vi "limelightDrive.vi"(10 "reinitialize? (F)":bool) -> (0 "Valid Track":bool=TRUE, 2 "Turn Output":dbl=0.011269776979651982)   [LabVIEW 2018]
uses:
  <vilib>/addons/control/pid/pid.llb/PID (DBL).vi
  <vilib>/addons/control/pid/NI_PID_pid.lvlib
panel:
  in  "output range":cluster{"output high":dbl, "output low":dbl}={"output high"=0.6, "output low"=-0.6}
  out "PID Output":dbl(graph)=0.011269776979651982
  in  "PID gains":T1={"proportional gain (Kc)"=0.013, "integral time (Ti, min)"=0.2, "derivative time (Td, min)"=0.0009} {"derivative time (Td, min)" format="%.4f"; "integral time (Ti, min)" format="%.3f"; "proportional gain (Kc)" format="%.3f"}
  out "Camera X":cluster{"setpoint":dbl, "Double":dbl}(graph)={"setpoint"=0.0, "Double"=-0.6907806396484375}
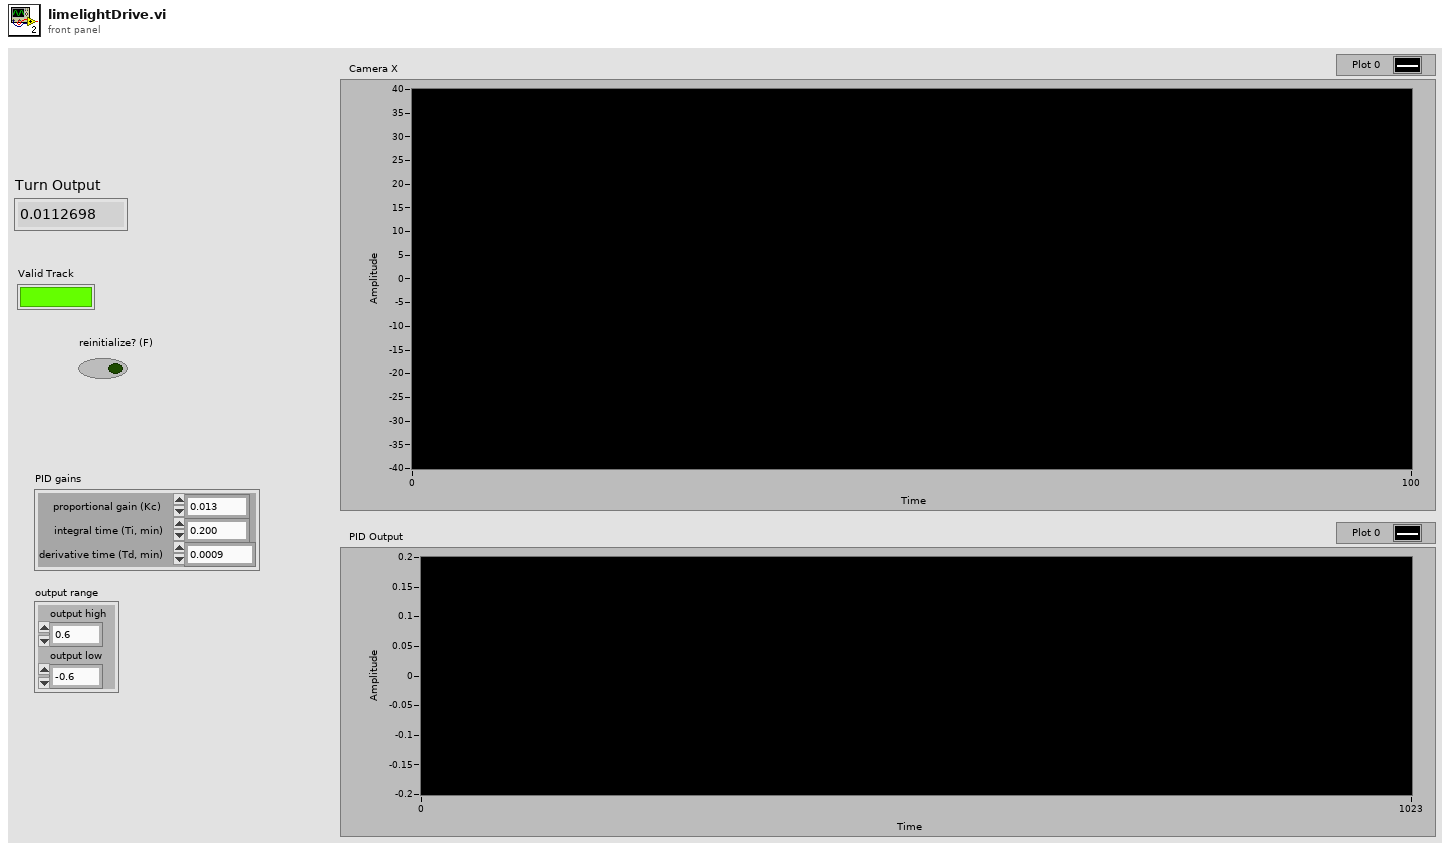
[diagram p1: front panel]
types:
  T1 = cluster{"proportional gain (Kc)":dbl, "integral time (Ti, min)":dbl, "derivative time (Td, min)":dbl}
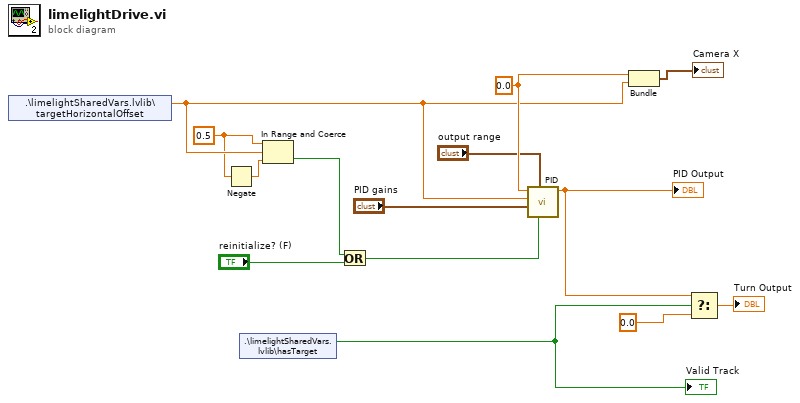
[diagram p0: block diagram]
diagram:
  w6 = 0.5 ("upper limit")
  w14 = 0.0 ("setpoint")
  n1 = shared-variable ".\\limelightSharedVars.lvlib\\targetHorizontalOffset"() -> (w8:dbl)  [unwired: 1 in, 1 out]
  n2 = Negate(x=w6) -> (-x=w7:dbl)
  n3 = shared-variable ".\\limelightSharedVars.lvlib\\hasTarget"() -> (w2:bool)  [unwired: 1 in, 1 out]
  "Valid Track" <- w2
  n4 = In Range and Coerce(upper limit=w6, x=w8, lower limit=w7) -> (In Range?=w3:bool)  [unwired: 1 out]
  n5 = Or(x=w3, y="reinitialize? (F)") -> (x .or. y?=w5:bool)
  n6 = call-poly <vilib>:"PID.vi"("reinitialize? (F)"=w5, "output range"="output range", "PID gains"="PID gains", "process variable"=w8, "setpoint"=w14) -> ("output"=w12:dbl)  [unwired: 5 in, 1 out]
  "PID Output" <- w12
  n7 = Bundle("setpoint"=w14, "Double"=w8) -> (→"Camera X":cluster{"setpoint":dbl, "Double":dbl})  [unwired: 1 in]
  n8 = Select(t=w12, s=w2, f=0.0) -> (s? t:f=→"Turn Output":dbl)
